vi "Update analysis parameters.vi"(6 "wait for reply (T)":bool=TRUE, 7 "Savitzksky-Golay":T1={"Sidepoints (M)"=20.0, "Filter Order"=5} {"Filter Order" scale=0.0..10.0; "Sidepoints (M)" scale=0.0..10.0}, 8 "error in":errorcluster, 9 "Decimation":T2={"App"={"Dec"=1, "apply"=FALSE}, "Con"={"Dec"=1, "apply"=FALSE}, "Ret"={"Dec"=1, "apply"=FALSE}}, 10 "Contact":T3={"Contact stat?"=TRUE, "Contact Spread of dev"=0.0} {"Contact Spread of dev" format="%#_13g"}) -> (0 "error out":errorcluster, 1 "timed out?":bool, 3 "updated":bool)   [LabVIEW 2019, in "Analysis.lvlib"]
doc: "Updates the analsysis parameters\n_____\nCreated using DQMH Event Scripter 6.1.0.128."
uses:
  Analysis.lvlib
  Main UI Shared/Decimation input --cluster.ctl
  Update analysis parameters Argument--cluster.ctl
  Update analysis parameters (Reply Payload)--cluster.ctl
  Main UI Shared/MAIN UI Shared.lvlib
panel:
  # "Contact"
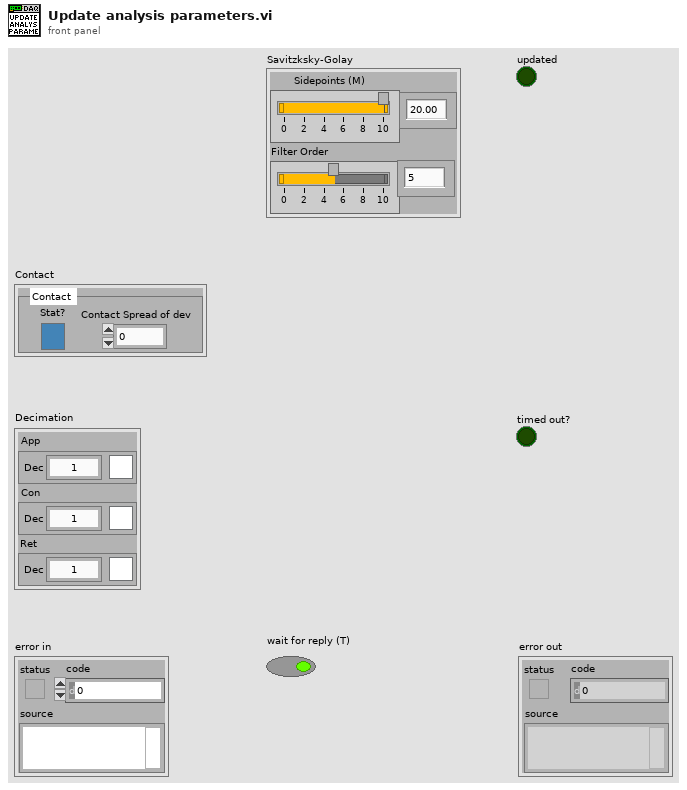
[diagram p1: front panel]
types:
  T1 = cluster{"Sidepoints (M)":dbl, "Filter Order":i32}
  T2 = typedef "MAIN UI Shared.lvlib/Decimation input --cluster.ctl" = cluster{"App":cluster{"Dec":i32, "apply":bool}, "Con":cluster{"Dec":i32, "apply":bool}, "Ret":cluster{"Dec":i32, "apply":bool}}
  T3 = cluster{"Contact stat?":bool, "Contact Spread of dev":dbl}
  T4 = typedef "Analysis.lvlib/Update analysis parameters Argument--cluster.ctl" = cluster{"Contact":cluster{"Contact stat?":bool, "Contact Spread of dev":dbl}, "Decimation":T2, "Savitzksky-Golay":cluster{"Sidepoints (M)":dbl, "Filter Order":i32}, "Wait Notifier":refnum<notifier>, "wait for reply":bool}
  T5 = typedef "Analysis.lvlib/Request Events--cluster.ctl" = cluster{"Stop Module":refnum<user-event>, "Show Panel":refnum<user-event>, "Hide Panel":refnum<user-event>, "Get Module Execution Status":refnum<user-event>, "Show Diagram":refnum<user-event>, "Wakeup Helper Loop":refnum<user-event>, "Change Settings":refnum<user-event>, "Update analysis parameters":refnum<user-event>, "Update Savitzky parameters":refnum<user-event>, "Update decimation":refnum<user-event>, "Update contact parameters":refnum<user-event>, "Update Tau delay (ms)":refnum<user-event>, "Open Fcurve object":refnum<user-event>, "Apply Savitzky Golay Filter":refnum<user-event>, "Apply decimation":refnum<user-event>}
  T6 = typedef "Analysis.lvlib/Update analysis parameters (Reply Payload)--cluster.ctl" = cluster{"updated":bool, "error":errorcluster}
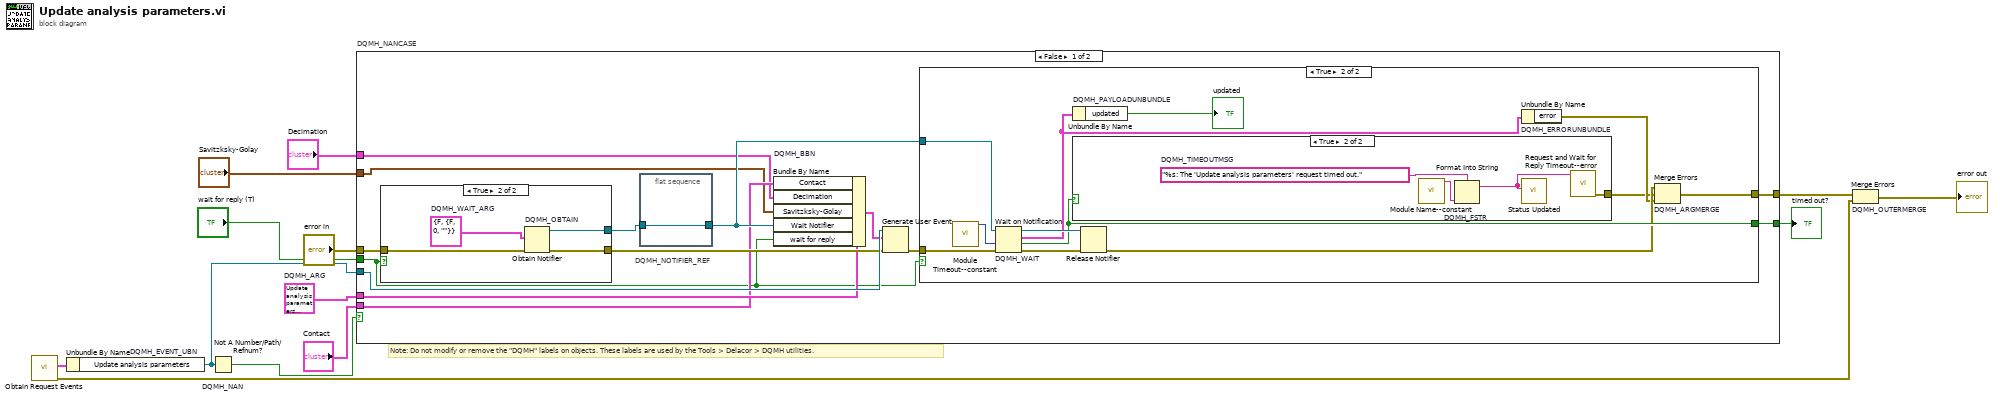
[diagram p0: block diagram]
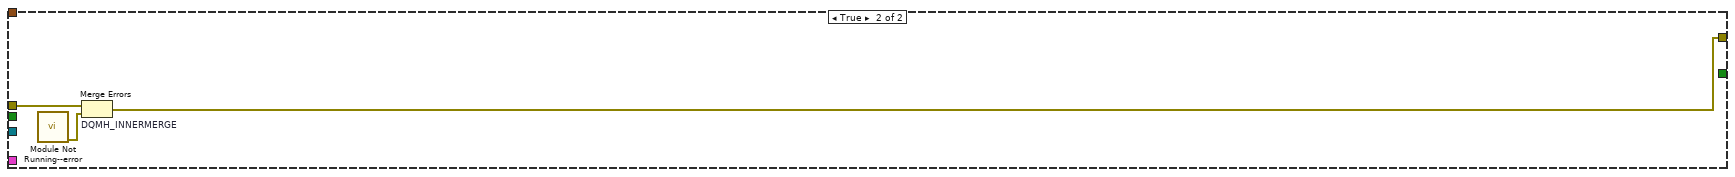
[diagram p5: hidden frame]
diagram:
  w7 = T4 {"Contact"={"Contact stat?"=TRUE, "Contact Spread of dev"=0.0}, "Decimation"={"App"={"Dec"=1, "apply"=FALSE}, "Con"={"Dec"=1, "apply"=FALSE}, "Ret"={"Dec"=1, "apply"=FALSE}}, "Savitzksky-Golay"={"Sidepoints (M)"=20.0, "Filter Order"=5}, "Wait Notifier"=refnum, "wait for reply"=FALSE}  # DQMH_ARG
  # "Note: Do not modify or remove the \"DQMH\" labels on objects. These labels are used by the Tools > Delacor > DQMH utilities."
  n1 = call "Obtain Request Events.vi"() -> ("error out"=w2:errorcluster, "Analysis Request Events"=w1:T5)  [unwired: 10 in]
  n2 = Unbundle By Name "DQMH_EVENT_UBN"(w1) -> ("Update analysis parameters"=w11:refnum<user-event>)
  n3 = Not A Number/Path/Refnum? "DQMH_NAN"(number/path/refnum=w11) -> (NaN/Path/Refnum?=w10:bool)
  n4 = case "DQMH_NANCASE" shown="False" w10 {
    tunnel: "error in" -> [w27 w53]
    tunnel: w11 -> [w25 _]
    tunnel: [w22 w52] -> w8
    tunnel: [w23 _] -> w9
    tunnel: w7 -> [w18 _]
    tunnel: "Contact" -> [w17 _]
    tunnel: "Decimation" -> [w16 _]
    tunnel: "Savitzksky-Golay" -> [w15 _]
    tunnel: "wait for reply (T)" -> [w14 _]
    frame False {
      n5 = case shown="True" w14 {
        tunnel: w27 -> [w46 w50]
        tunnel: [w46 w49] -> w24
        tunnel: [_ w47] -> w20
        frame False {
        }
        frame True {
          w48 = T6 {"updated"=FALSE, "error"={"status"=FALSE, "code"=0, "source"=""}}  # DQMH_WAIT_ARG
          n6 = Obtain Notifier "DQMH_OBTAIN"(notification data type=w48, error in (no error)=w50) -> (notifier out=w47:refnum<notifier>, error out=w49:errorcluster)  [unwired: 2 in, 1 out]
        }
      }
      n7 = flat-sequence "DQMH_NOTIFIER_REF" {
        tunnel: w20 -> [w28]
        tunnel: [w28] -> w19
        frame #0 {
        }
      }
      n8 = Bundle By Name "DQMH_BBN"(cluster=w18, "Contact"=w17, "Decimation"=w16, "Savitzksky-Golay"=w15, "Wait Notifier"=w19, "wait for reply"=w14) -> (w21:T4)
      n9 = Generate User Event(user event=w25, event data cluster=w21, error in=w24) -> (error out=w26:errorcluster)  [unwired: 1 in, 1 out]
      n10 = case shown="True" w14 {
        tunnel: w26 -> [w29 w41]
        tunnel: w19 -> [_ w40]
        tunnel: [_ w38] -> w23
        tunnel: [w29 w37] -> w22
        frame False {
        }
        frame True {
          n11 = call "Module Timeout--constant.vi"() -> ("Module Timeout"=w31:i32)  [unwired: 11 in]
          n12 = Wait on Notification "DQMH_WAIT"(notifier=w40, timeout in ms (-1)=w31, error in (no error)=w41) -> (notifier out=w39:refnum<notifier>, notification=w32:T6, timed out?=w38:bool, error out=w36:errorcluster)  [unwired: 1 in]
          n13 = Unbundle By Name "DQMH_PAYLOADUNBUNDLE"(w32) -> ("updated"=→"updated":bool)
          n14 = case shown="True" w38 {
            tunnel: [_ w43] -> w33
            frame False {
            }
            frame True {
              w45 = "%s: The 'Update analysis parameters' request timed out."  # DQMH_TIMEOUTMSG
              n15 = call "Module Name--constant.vi"() -> ("Module Name"=w42:string)  [unwired: 11 in]
              n16 = Format Into String "DQMH_FSTR"(format string=w45, w42) -> (resulting string=w44:string)  [unwired: 2 in, 1 out]
              n17 = call "Status Updated.vi"("Status"=w44) -> ()  [unwired: 10 in, 1 out]
              n18 = call "Request and Wait for Reply Timeout--error.vi"("Error Message"=w44) -> ("error out"=w43:errorcluster)  [unwired: 10 in]
            }
          }
          n19 = Release Notifier(notifier=w39, error in (no error)=w36) -> (error out=w35:errorcluster)  [unwired: 1 in, 2 out]
          n20 = Unbundle By Name "DQMH_ERRORUNBUNDLE"(w32) -> ("error"=w34:errorcluster)
          n21 = Merge Errors "DQMH_ARGMERGE"(w35, w33, w34) -> (w37:errorcluster)
        }
      }
    }
    frame True {
      n22 = call "Module Not Running--error.vi"() -> ("error out"=w51:errorcluster)  [unwired: 11 in]
      n23 = Merge Errors "DQMH_INNERMERGE"(w53, w51) -> (w52:errorcluster)
    }
  }
  "timed out?" <- w9
  n24 = Merge Errors "DQMH_OUTERMERGE"(w8, w2) -> (→"error out":errorcluster)
